vi "WSVCAP SHL FPGA LL RFFE Set Data Enable State.vi"(0 "State":bool, 11 "error in (no error)":errorcluster) -> (15 "error out":errorcluster)   [LabVIEW 2012]
uses:
  <vilib>/eio/EIOMethodNode/EIOMethodNode.xnode
  <vilib>/rvi/eio/common/nirviEmuTemplateMethod_errors.vi
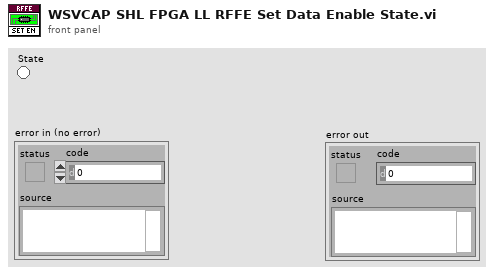
[diagram p1: front panel]
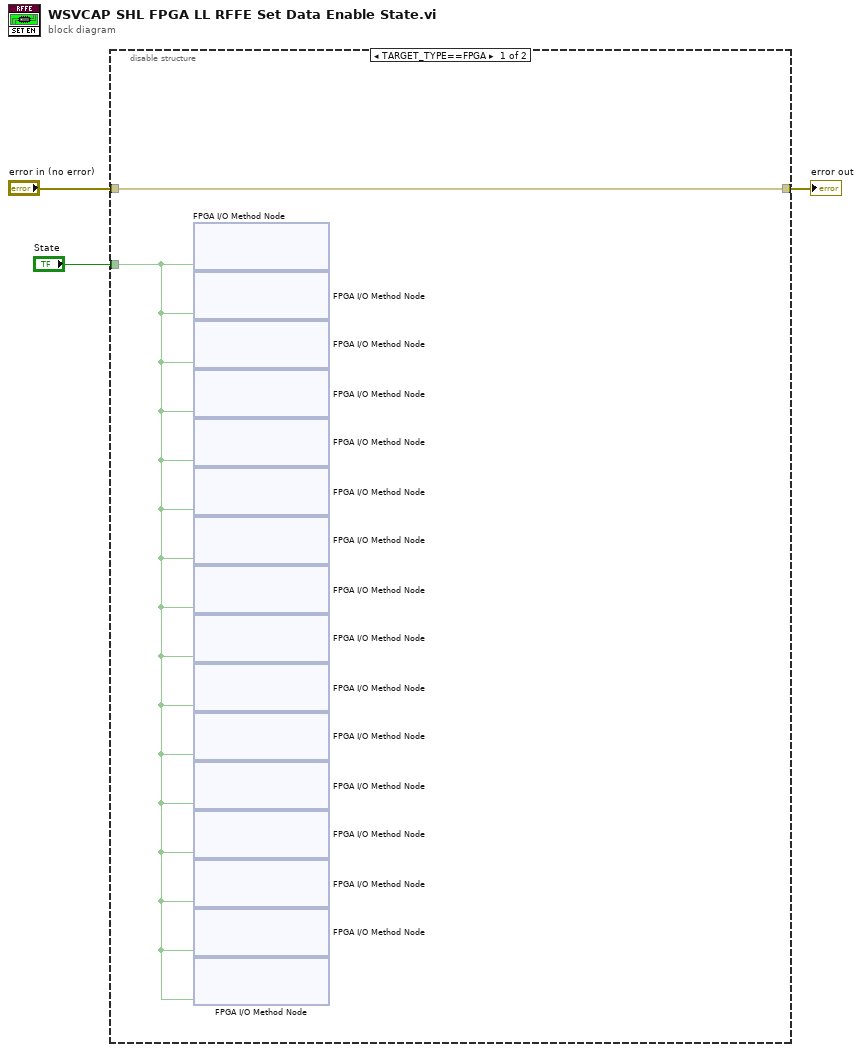
[diagram p0: block diagram]
diagram:
  n1 = disable-structure shown="TARGET_TYPE==FPGA" {
    disable-tunnel: "State" -> [w4 _]
    disable-tunnel: [w5 w6] -> w2
    disable-tunnel: "error in (no error)" -> [w5 w6]
    frame condition #0 {
      n2 = xnode "FPGA I/O Method Node"("Enable"=w4) -> ()  [unwired: 1 in, 1 out]
      n3 = xnode "FPGA I/O Method Node"("Enable"=w4) -> ()  [unwired: 1 in, 1 out]
      n4 = xnode "FPGA I/O Method Node"("Enable"=w4) -> ()  [unwired: 1 in, 1 out]
      n5 = xnode "FPGA I/O Method Node"("Enable"=w4) -> ()  [unwired: 1 in, 1 out]
      n6 = xnode "FPGA I/O Method Node"("Enable"=w4) -> ()  [unwired: 1 in, 1 out]
      n7 = xnode "FPGA I/O Method Node"("Enable"=w4) -> ()  [unwired: 1 in, 1 out]
      n8 = xnode "FPGA I/O Method Node"("Enable"=w4) -> ()  [unwired: 1 in, 1 out]
      n9 = xnode "FPGA I/O Method Node"("Enable"=w4) -> ()  [unwired: 1 in, 1 out]
      n10 = xnode "FPGA I/O Method Node"("Enable"=w4) -> ()  [unwired: 1 in, 1 out]
      n11 = xnode "FPGA I/O Method Node"("Enable"=w4) -> ()  [unwired: 1 in, 1 out]
      n12 = xnode "FPGA I/O Method Node"("Enable"=w4) -> ()  [unwired: 1 in, 1 out]
      n13 = xnode "FPGA I/O Method Node"("Enable"=w4) -> ()  [unwired: 1 in, 1 out]
      n14 = xnode "FPGA I/O Method Node"("Enable"=w4) -> ()  [unwired: 1 in, 1 out]
      n15 = xnode "FPGA I/O Method Node"("Enable"=w4) -> ()  [unwired: 1 in, 1 out]
      n16 = xnode "FPGA I/O Method Node"("Enable"=w4) -> ()  [unwired: 1 in, 1 out]
      n17 = xnode "FPGA I/O Method Node"("Enable"=w4) -> ()  [unwired: 1 in, 1 out]
    }
    frame condition #1 (active) {
    }
  }
  "error out" <- w2
